vi "CompressCircle - Kibble-Zurek.vi"(6 "Steps":u32, 8 "R0":dbl, 9 "Delta R":dbl, 10 "Time":dbl, 11 "input ellipse params":T1={"Radius"=0.0, "No. of Points"=0, "Center"={"X"=0.0, "Y"=0.0}, "Circle"=FALSE, "Density"=0.0, "PointSpec"=enum."No. Of Points", "Hold"=FALSE, "Size"=1, "LatC"=10.0, "Eccentricity"=0.0, "Phase"=0.0} {"Eccentricity" min=0.0; "Size" step=1; "LatC" step=0.05}) -> (3 "output ellipse params":T1={"Radius"=0.0, "No. of Points"=0, "Center"={"X"=0.0, "Y"=0.0}, "Circle"=FALSE, "Density"=0.0, "PointSpec"=enum."No. Of Points", "Hold"=FALSE, "Size"=1, "LatC"=10.0, "Eccentricity"=0.0, "Phase"=0.0} {"Eccentricity" min=0.0; "Size" step=1; "LatC" step=0.05})   [LabVIEW 2017]
uses:
  CircleControls.ctl
  AODControl/AODGlobals.vi
  AODControl/MessageQueue/QueueOperations/Enqueue Message (Single).vi
  AODControl/MessageQueue/MessageQueue.lvlib
  AODControl/AODControl.lvlib
panel:
  out "Current Radius":dbl
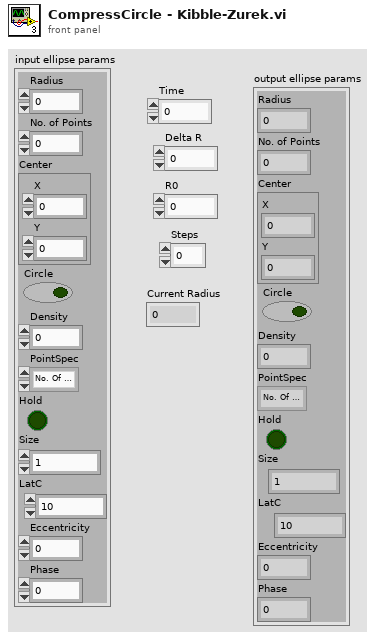
[diagram p1: front panel]
types:
  T1 = typedef "CircleControls.ctl" = cluster{"Radius":dbl, "No. of Points":i32, "Center":cluster{"X":dbl, "Y":dbl}, "Circle":bool, "Density":dbl, "PointSpec":enum32{"No. Of Points", "Density"}, "Hold":bool, "Size":i32, "LatC":dbl, "Eccentricity":dbl, "Phase":dbl}
  T2 = typedef "AODControl.lvlib/MessageQueue.lvlib/All Message Queues.ctl" = cluster{" AOD Interface":refnum<queue>}
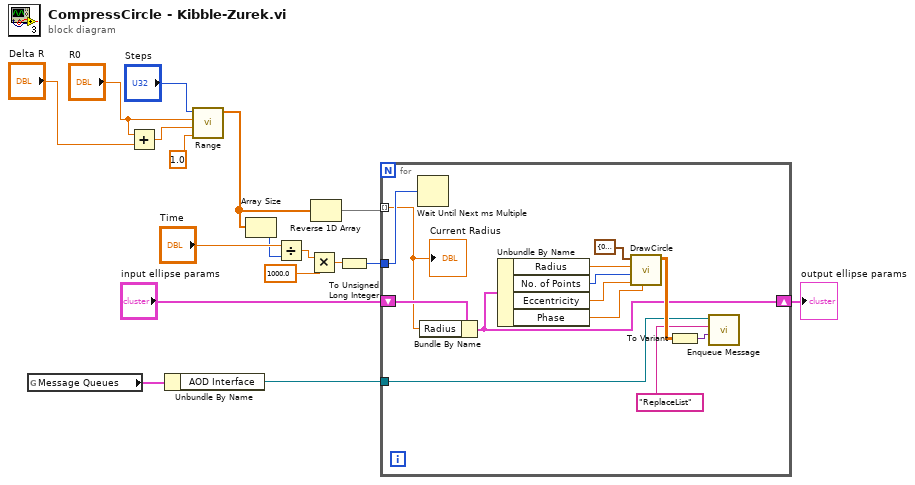
[diagram p0: block diagram]
diagram:
  n1 = global read "AODGlobals.vi" "Message Queues"() -> (w16:T2)
  n2 = Add(x="R0", y="Delta R") -> (x+y=w11:dbl)
  n3 = Unbundle By Name(w16) -> ("AOD Interface"=w15:refnum<queue>)
  n4 = call "Range.vi"("Exponent"=1.0, "End"=w11, "Start"="R0", "Steps"="Steps") -> ("Array"=w3:dbl[])  [unwired: 7 in]
  n5 = Array Size(array=w3) -> (size(s)=w5:i32)
  n6 = Divide(x="Time", y=w5) -> (x/y=w9:dbl)
  n7 = Multiply(x=w9, y=1000.0) -> (x*y=w7:dbl)
  n8 = Reverse 1D Array(array=w3) -> (reversed array=w4:dbl[])
  n9 = To Unsigned Long Integer(number=w7) -> (unsigned 32bit integer=w6:u32)
  n10 = for {
    tunnel: w15 -> [w26]
    tunnel: w4 -> [w20] mode=indexing
    tunnel: w6 -> [w22]
    shift-right: [w18] -> w2
    shift-left: "input ellipse params" -> [w21]
    n11 = Wait Until Next ms Multiple(millisecond multiple=w22) -> ()  [unwired: 1 out]
    n12 = Bundle By Name(cluster=w21, "Radius"=w20) -> (w18:T1)
    n13 = Unbundle By Name(w18) -> ("Radius"=w19:dbl, "No. of Points"=w29:i32, "Eccentricity"=w24:dbl, "Phase"=w23:dbl)
    n14 = call "DrawCircle.vi"("Phase"=w23, "Eccentricity"=w24, "No Of Points"=w29, "Radius"=w19, "Center"=cluster{"X":dbl, "Y":dbl} {"X"=0.0, "Y"=0.0}) -> ("Array"=w28:dbl[][])  [unwired: 6 in]
    n15 = To Variant(anything=w28) -> (Variant=w30:variant)
    n16 = call-poly "Enqueue Message.vi"("Message Data"=w30, "Message"="ReplaceList", "Message Queue"=w26) -> ()  [unwired: 7 in, 2 out]
    "Current Radius" <- w20
  }
  "output ellipse params" <- w2
